vi "Test FPGA.vi"() -> ()   [LabVIEW 2016]
uses:
  <vilib>/rvi/interface/RandomDataEmulation/nirviRandomDataOpen.vi
  <vilib>/rvi/interface/RandomDataEmulation/nirviRandomDataDMAMethods.vi
  <vilib>/rvi/interface/nirviOpenFPGA/nirviOpenFPGA.xnode
  <vilib>/rvi/interface/nirviMethod/nirviMethod.xnode
panel:
  out "error out":errorcluster
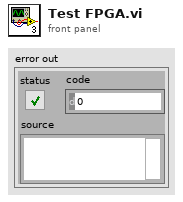
[diagram p1: front panel]
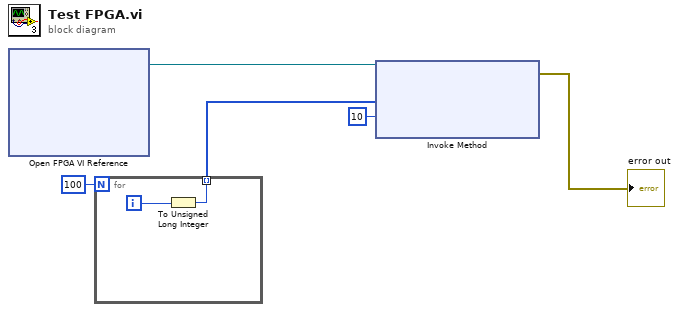
[diagram p0: block diagram]
diagram:
  n1 = xnode "Open FPGA VI Reference"() -> ("FPGA VI Reference Out"=w5:refnum<k20>)  [unwired: 2 in, 1 out]
  n2 = for {
    N: 100 -> [_]
    tunnel: [w7] -> w3 mode=indexing
    i -> [w6]
    n3 = To Unsigned Long Integer(number=w6) -> (unsigned 32bit integer=w7:u32)
  }
  n4 = xnode "Invoke Method"("FPGA VI Reference In"=w5, "Data"=w3, "Timeout (ms)"=10) -> ("error out"=→"error out":errorcluster)  [unwired: 1 in, 2 out]
